vi "controlespejolito.vi"(4 "y inicial":dbl, 6 "x inicial":dbl, 8 "intervalo y":dbl, 9 "intervalo x":dbl, 10 "cadena entrada":string) -> (1 "x":dbl, 2 "y":dbl)   [LabVIEW 2016]
doc: "Este subVI recibe los datos de la posición del spot en una cadena, los convierte a número flotante y los envia al ni cRIO para poder mover los espejos.\n\nComo entradas están:\n\nLa cadena que contiene los valors de voltaje para mover los espejos.\n\nComo salidas están los valores en x y y de los voltajes aplicados a los espejos."
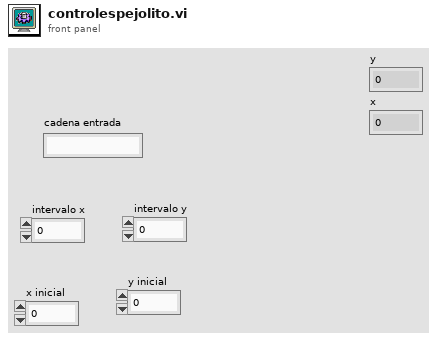
[diagram p1: front panel]
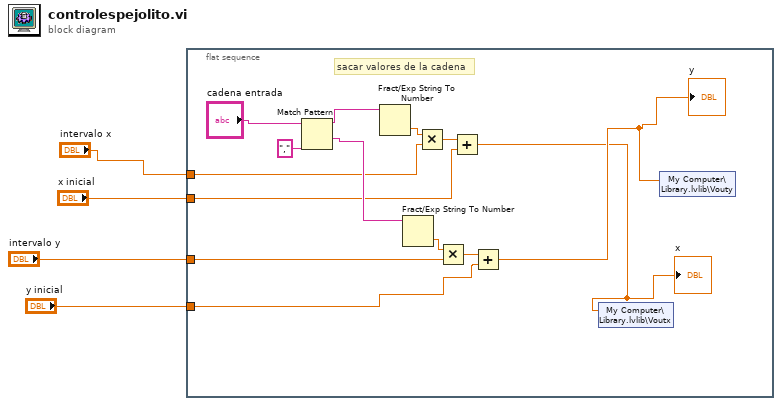
[diagram p0: block diagram]
diagram:
  n1 = flat-sequence {
    tunnel: "intervalo y" -> [w13]
    tunnel: "y inicial" -> [w11]
    tunnel: "intervalo x" -> [w7]
    tunnel: "x inicial" -> [w6]
    frame #0 {
      # "sacar valores de la cadena"
      n2 = Match Pattern(string="cadena entrada", regular expression=",") -> (before substring=w16:string, after substring=w15:string)  [unwired: 1 in, 2 out]
      n3 = Fract/Exp String To Number(string=w16) -> (number=w8:dbl)  [unwired: 3 in, 1 out]
      n4 = Fract/Exp String To Number(string=w15) -> (number=w14:dbl)  [unwired: 3 in, 1 out]
      n5 = Multiply(x=w8, y=w7) -> (x*y=w9:dbl)
      n6 = Multiply(x=w14, y=w13) -> (x*y=w12:dbl)
      n7 = Add(x=w9, y=w6) -> (x+y=w5:dbl)
      "x" <- w5
      n8 = Add(x=w12, y=w11) -> (x+y=w10:dbl)
      "y" <- w10
      n9 = shared-variable "My Computer\\Library.lvlib\\Voutx"(w5) -> ()  [unwired: 1 in, 1 out]
      n10 = shared-variable "My Computer\\Library.lvlib\\Vouty"(w10) -> ()  [unwired: 1 in, 1 out]
    }
  }
